vi "checksum_i.vi"(10 "check dataName":string, 11 "string":string) -> (2 "Boolean":bool, 3 "String":string)   [LabVIEW 2020]
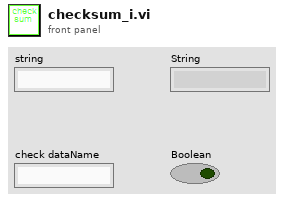
[diagram p1: front panel]
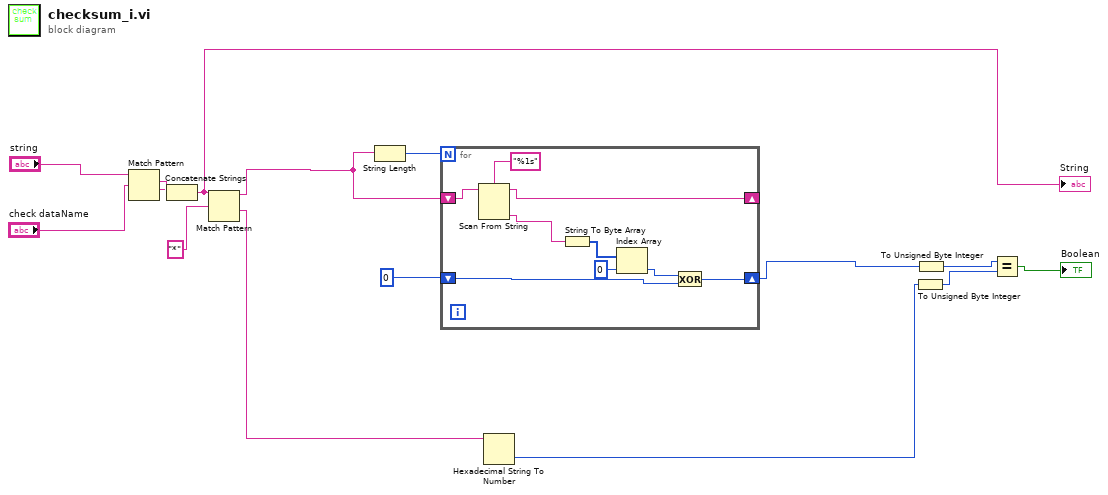
[diagram p0: block diagram]
diagram:
  n1 = Match Pattern(string="string", regular expression="check dataName") -> (match substring=w14:string, after substring=w13:string)  [unwired: 1 in, 2 out]
  n2 = Concatenate Strings(w14, w13) -> (w5:string)
  "String" <- w5
  n3 = Match Pattern(string=w5, regular expression="*") -> (before substring=w2:string, after substring=w10:string)  [unwired: 1 in, 2 out]
  n4 = String Length(string=w2) -> (length=w4:i32)
  n5 = for {
    N: w4 -> [_]
    shift-right: [w17] -> _
    shift-left: w2 -> [w23]
    shift-right: [w18] -> w1
    shift-left: u8 0 -> [w19]
    n6 = Scan From String(format string="%1s", input string=w23) -> (remaining string=w17:string, output 1=w16:string)  [unwired: 3 in, 2 out]
    n7 = String To Byte Array(string=w16) -> (unsigned byte array=w22:u8[])
    n8 = Index Array(array=w22, index=0) -> (element=w20:u8)
    n9 = Exclusive Or(1:w19, 2:w20) -> (0:w18:u8)
  }
  n10 = Hexadecimal String To Number(string=w10) -> (number=w9:u32)  [unwired: 2 in, 1 out]
  n11 = To Unsigned Byte Integer(number=w9) -> (unsigned 8bit integer=w8:u8)
  n12 = To Unsigned Byte Integer(number=w1) -> (unsigned 8bit integer=w7:u8)
  n13 = Equal?(x=w7, y=w8) -> (x = y?=→"Boolean":bool)
